vi "Read Trace.vi"(8 "error in (no error)":errorcluster, 9 "Maximum Time (10000)":u32=10000, 11 "VISA resource name":refnum<visa-resource-name>) -> (0 "error out":errorcluster, 3 "VISA resource name out":refnum<visa-resource-name>, 5 "Y array":dbl[](array[numeric]), 7 "X array":dbl[](array[numeric]))   [LabVIEW 2021, in "Ceyear.lvlib"]
doc: "Reads a trace from the spectrum analyzer."
uses:
  <instrlib>/Ceyear/Ceyear.lvlib
panel:
  out "XY Graph":cluster{"X array":dbl[], "Y array":dbl[]}(graph)
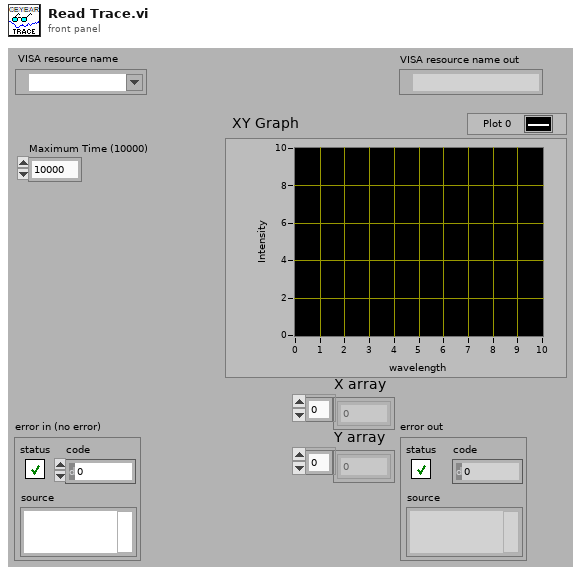
[diagram p1: front panel]
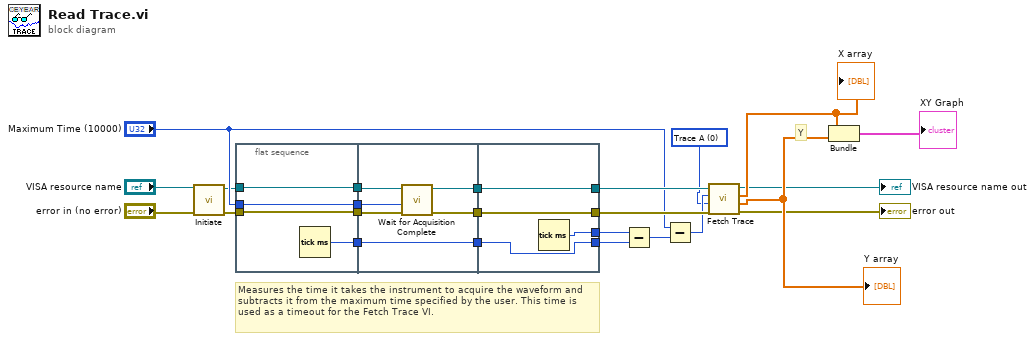
[diagram p0: block diagram]
diagram:
  w10 = u16 0 items=["Trace A", "Trace B", "Trace C", "Trace D", "Trace E"] ("Ring")
  # "Measures the time it takes the instrument to acquire the waveform and subtracts it from the maximum time specified by the user. This time is used as a timeout for the Fetch Trace VI."
  # "Y"
  n1 = call <instrlib>:"Initiate.vi"("error in (no error)"="error in (no error)", "VISA resource name"="VISA resource name") -> ("error out"=w5:errorcluster, "VISA resource name out"=w6:refnum<visa-resource-name>)  [unwired: 8 in]
  n2 = flat-sequence {
    tunnel: [w28] -> w18
    tunnel: w6 -> [w27]
    tunnel: [w27] -> w17
    tunnel: w5 -> [w26]
    tunnel: [w26] -> w16
    tunnel: "Maximum Time (10000)" -> [w25]
    tunnel: [w25] -> w15
    tunnel: w18 -> [w29]
    tunnel: [w29] -> w14
    tunnel: w17 -> [w34]
    tunnel: [w33] -> w13
    tunnel: w16 -> [w32]
    tunnel: [w31] -> w12
    tunnel: w15 -> [w30]
    tunnel: [w37] -> w23
    tunnel: w14 -> [w37]
    tunnel: [w38] -> w22
    tunnel: [w36] -> w21
    tunnel: w13 -> [w36]
    tunnel: [w35] -> w20
    tunnel: w12 -> [w35]
    frame #0 {
      n3 = Tick Count (ms)() -> (millisecond timer value=w28:u32)
    }
    frame #1 {
      n4 = call <instrlib>:"Wait for Acquisition Complete.vi"("error in (no error)"=w32, "Maximum Time (10000)"=w30, "VISA resource name"=w34) -> ("error out"=w31:errorcluster, "VISA resource name out"=w33:refnum<visa-resource-name>)  [unwired: 7 in]
    }
    frame #2 {
      n5 = Tick Count (ms)() -> (millisecond timer value=w38:u32)
    }
  }
  n6 = Subtract(x=w22, y=w23) -> (x-y=w24:u32)
  n7 = Subtract(x="Maximum Time (10000)", y=w24) -> (x-y=w11:u32)
  n8 = call <instrlib>:"Fetch Trace.vi"("error in (no error)"=w20, "Trace"=w10, "Maximum time"=w11, "VISA resource name"=w21) -> ("error out"=→"error out":errorcluster, "Y array"=w9:dbl[], "X array"=w8:dbl[], "VISA resource name out"=→"VISA resource name out":refnum<visa-resource-name>)  [unwired: 4 in]
  "X array" <- w8
  "Y array" <- w9
  n9 = Bundle("X array"=w8, "Y array"=w9) -> (→"XY Graph":cluster{"X array":dbl[], "Y array":dbl[]})  [unwired: 1 in]
